vi "MDAQ_CaptureTemps.vi"(9 "Main Cluster":T1 {"CV"."Temperature Array" scale=0.0..100.0}, 10 "Status Cluster":T3 {"GATESTOP" format="%04x"; "GATESTRT" format="%04x"; "AMPLITUDE" format="%04x"; "M_CYCLES" format="%04x"; "N_CYCLES" format="%04x"; "STEP" format="%04x"; "BASE" format="%04x"; "CHAN" format="%04x"}) -> (1 "Main Cluster Out":T1 {"CV"."Temperature Array" scale=0.0..100.0}, 2 "Status Cluster Out":T3 {"GATESTOP" format="%04x"; "GATESTRT" format="%04x"; "AMPLITUDE" format="%04x"; "M_CYCLES" format="%04x"; "N_CYCLES" format="%04x"; "STEP" format="%04x"; "BASE" format="%04x"; "CHAN" format="%04x"})   [LabVIEW 2021]
uses:
  Status_Cluster.ctl
  GUI_Def.ctl
  Mode_Enum.ctl
  <vilib>/Analysis/baseanly.llb/Mean (DBL).vi
  <vilib>/Analysis/NI_AALBase.lvlib
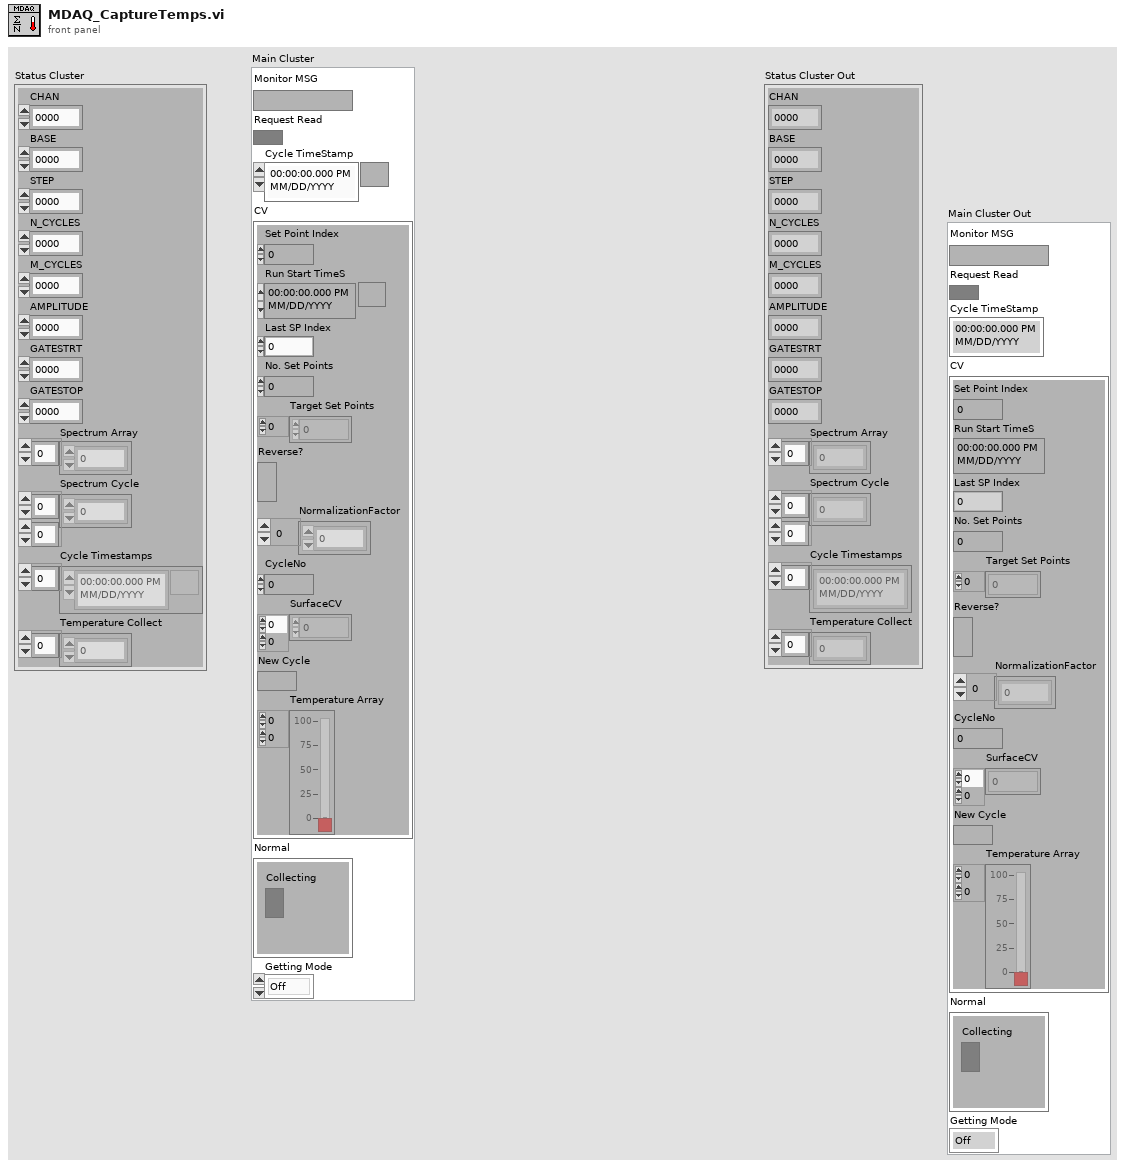
[diagram p1: front panel]
types:
  T1 = typedef "GUI_Def.ctl" = cluster{"Monitor MSG":string, "Request Read":bool, "Cycle TimeStamp":timestamp, "CV":cluster{"Set Point Index":u32, "Run Start TimeS":timestamp, "Last SP Index":u32, "No. Set Points":u32, "Target Set Points":i32[], "Reverse?":bool, "NormalizationFactor":i32[], "CycleNo":i32, "SurfaceCV":dbl[][], "New Cycle":bool, "Temperature Array":dbl[][]}, "Normal":cluster{"Collecting":bool}, "Getting Mode":T2}
  T2 = typedef "Mode_Enum.ctl" = enum16{"Off", "Normal", "CV+Temp", "CV"}
  T3 = typedef "Status_Cluster.ctl" = cluster{"CHAN":u32, "BASE":u32, "STEP":u32, "N_CYCLES":u32, "M_CYCLES":u32, "AMPLITUDE":u32, "GATESTRT":u32, "GATESTOP":u32, "Spectrum Array":u32[], "Spectrum Cycle":u32[][], "Cycle Timestamps":timestamp[], "Temperature Collect":dbl[]}
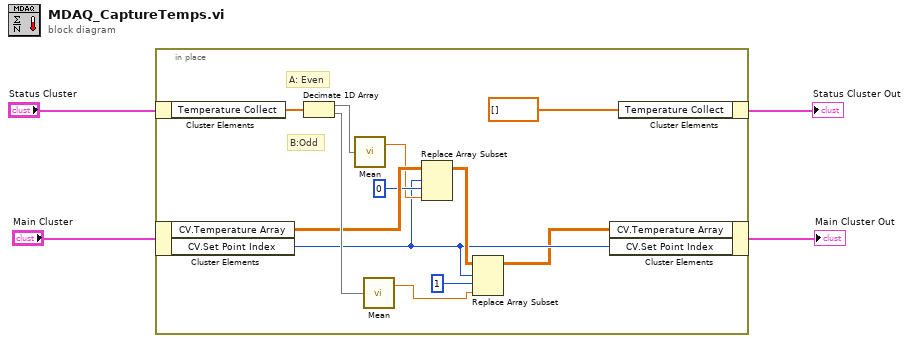
[diagram p0: block diagram]
diagram:
  n1 = in-place {
    # "B:Odd"
    # "A: Even"
    n2 = in-place-cluster #1("Status Cluster") -> ("Temperature Collect"=w16:dbl[])
    n3 = in-place-cluster #2("Main Cluster") -> ("CV.Temperature Array"=w12:dbl[][], "CV.Set Point Index"=w8:u32)
    n4 = Decimate 1D Array(w16) -> (w14:dbl[], w13:dbl[])
    n5 = call-poly <vilib>:"Mean.vi"("X"=w14) -> ("mean"=w10:dbl)  [unwired: 1 out]
    n6 = call-poly <vilib>:"Mean.vi"("X"=w13) -> ("mean"=w6:dbl)  [unwired: 1 out]
    n7 = Replace Array Subset(array=w12, new element=w10, index (row)=w8, index (col)=0 ("disabled index (col)")) -> (w9:dbl[][])
    n8 = Replace Array Subset(array=w9, new element=w6, index (row)=w8, index (col)=1 ("disabled index (col)")) -> (w5:dbl[][])
    n9 = in-place-cluster #2("CV.Temperature Array"=w5, "CV.Set Point Index"=w8) -> (→"Main Cluster Out":T1)
    n10 = in-place-cluster #1("Temperature Collect"=dbl[] []) -> (→"Status Cluster Out":T3)
  }
